vi "test status reporting enable disable.vi"() -> ()   [LabVIEW 2013, in "std eng tests.lvlib"]
uses:
  std eng tests.lvlib
  Configuration/Standard Engine Configuration.lvclass
  Configuration/Standard Engine Configuration.lvclass/Standard Engine Configuration.ctl
  Configuration/Find Module Specific Config.vi
  <vilib>/Utility/error.llb/Error Cluster From Error Code.vi
  <vilib>/NI/CEF/CEF_TreeControl/serializable configuration/NISE_CEF_serializable configuration.lvclass
panel:
  out "disable after 2x no err":errorcluster
  out "enable 2x error":errorcluster
  out "missing tag (err)":errorcluster
  out "basics OK":bool
  out "error out":errorcluster
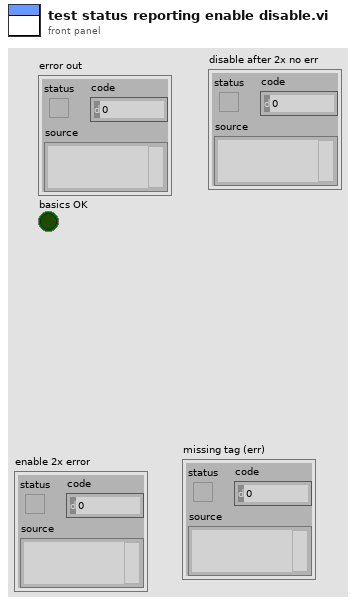
[diagram p1: front panel]
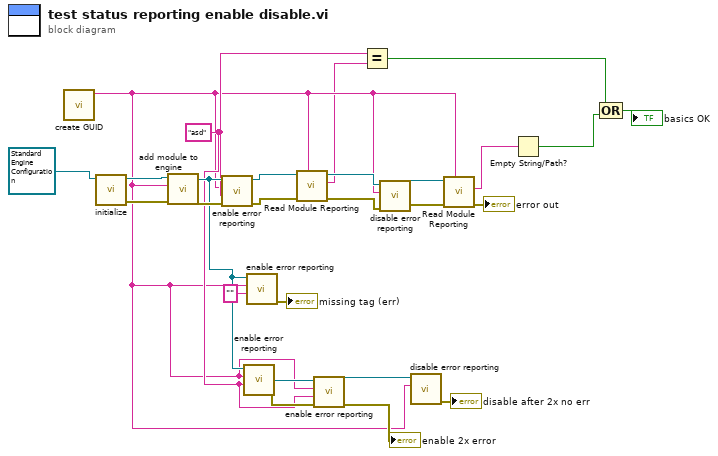
[diagram p0: block diagram]
diagram:
  w8 = "asd" ("tag")
  n1 = call <vilib>:"create GUID.vi"() -> ("uuid"=w4:string)  [unwired: 11 in]
  n2 = call-dynamic "initialize.vi"("configuration in"=refnum<class "Standard Engine Configuration.lvclass"> refnum ("Standard Engine Configuration")) -> ("error out"=w24:errorcluster, "configuration out"=w25:refnum<class "Standard Engine Configuration.lvclass">)  [unwired: 8 in, 1 out]
  n3 = call-dynamic "add module to engine.vi"("error in"=w24, "module ID"=w4, "Standard Engine Configuration in"=w25) -> ("error out"=w23:errorcluster, "Standard Engine Configuration out"=w9:refnum<class "Standard Engine Configuration.lvclass">)  [unwired: 7 in]
  n4 = call "enable error reporting.vi"("error in"=w23, "tag"=w8, "module ID"=w4, "Standard Engine Configuration in"=w9) -> ("error out"=w17:errorcluster, "Standard Engine Configuration out"=w20:refnum<class "Standard Engine Configuration.lvclass">)  [unwired: 6 in]
  n5 = call "enable error reporting.vi"("tag"=w8, "module ID"=w4, "Standard Engine Configuration in"=w9) -> ("error out"=w10:errorcluster, "Standard Engine Configuration out"=w11:refnum<class "Standard Engine Configuration.lvclass">)  [unwired: 7 in]
  n6 = call "enable error reporting.vi"("tag"="", "module ID"=w4, "Standard Engine Configuration in"=w9) -> ("error out"=→"missing tag (err)":errorcluster)  [unwired: 7 in, 1 out]
  n7 = call "Read Module Reporting.vi"("Module ID"=w4, "error in"=w17, "Standard Engine Repo Data in"=w20) -> ("error out"=w18:errorcluster, "error tag"=w2:string, "Standard Engine Repo Data out"=w19:refnum<class "Standard Engine Configuration.lvclass">)  [unwired: 6 in]
  n8 = call "enable error reporting.vi"("error in"=w10, "tag"=w8, "module ID"=w4, "Standard Engine Configuration in"=w11) -> ("error out"=→"enable 2x error":errorcluster, "Standard Engine Configuration out"=w5:refnum<class "Standard Engine Configuration.lvclass">)  [unwired: 6 in]
  n9 = Equal?(x=w8, y=w2) -> (x = y?=w15:bool)
  n10 = call "disable error reporting.vi"("error in"=w18, "module ID"=w4, "Standard Engine Configuration in"=w19) -> ("error out"=w21:errorcluster, "Standard Engine Configuration out"=w22:refnum<class "Standard Engine Configuration.lvclass">)  [unwired: 7 in]
  n11 = call "disable error reporting.vi"("module ID"=w4, "Standard Engine Configuration in"=w5) -> ("error out"=→"disable after 2x no err":errorcluster)  [unwired: 8 in, 1 out]
  n12 = call "Read Module Reporting.vi"("Module ID"=w4, "error in"=w21, "Standard Engine Repo Data in"=w22) -> ("error out"=→"error out":errorcluster, "error tag"=w1:string)  [unwired: 6 in, 1 out]
  n13 = Empty String/Path?(string/path=w1) -> (empty?=w16:bool)
  n14 = Compound Arithmetic op=OR(w15, w16) -> (→"basics OK":bool)
